vi "CANopencRIOPDODemo.vi"() -> ()   [LabVIEW 2016]
doc: "Write and Read PDO Values for PDO,1 which is mapped to digital values.\nThis example is written for a WAGO 750-307 device."
uses:
  <vilib>/Platform/TimedLoop/XDataNode/timing_clust.ctl
  <vilib>/Platform/TimedLoop/XDataNode/nitl_modes.ctl
  <vilib>/Platform/TimedLoop/XDataNode/wakeup.ctl
  Instance           2 26Saved   CANopencRIOPDODemo .vi
  Instance           3 26Saved   CANopencRIOPDODemo .vi
  <vilib>/FPGAPlugInAG/cRIO-9033/niLvFpga_Close_cRIO-9033.vi
  <vilib>/Platform/TimedLoop/XDataNode/XDataNode.xnode
  <vilib>/rvi/interface/nirviCloseFPGA/nirviCloseFPGA.xnode
  FPGA Bitfiles/EV-MCU_FPGATarget_CANEngine(FPGA)b_eM8Xz3qYJVA.lvbitx
  CAN_Engine(FPGA)_basic.vi
  <vilib>/Platform/TimedLoop/XDataNode/XDNodeRunTimeDep.lvlib
panel:
  out "ID":u32 format="%.0x"
  out "Finished Late? [i-1]":bool
  out "Timing (us)":u32
  out "error out":errorcluster
  in  "Digital Out":bool[](array[boolean])=[FALSE, FALSE, FALSE, FALSE, FALSE, FALSE, FALSE, FALSE, FALSE, FALSE, FALSE, FALSE, FALSE, FALSE, FALSE, FALSE]
  in  "stop":bool
  out "Digital In":bool[](array[boolean])
  # "Project uses 500 Kbaud\nand node ID 1"
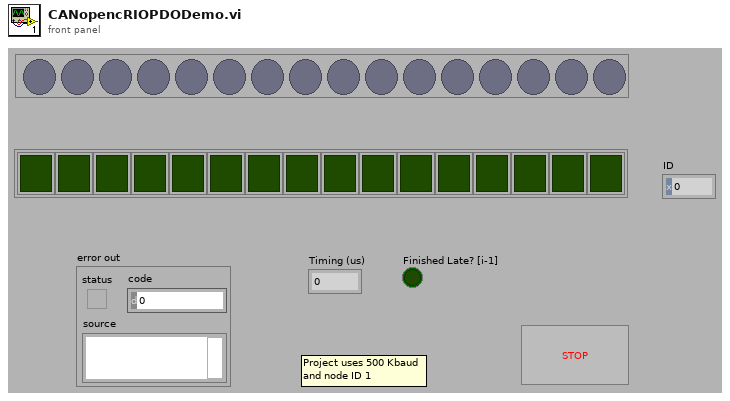
[diagram p1: front panel]
types:
  T1 = enum16{"start remote node", "stop remote node", "reset node", "reset communication", "enter preoperational"}
  T2 = typedef "XDNodeRunTimeDep.lvlib/timing_clust.ctl" = cluster{"Expected End [f-1]":u64, "Actual End [f-1]":u64, "Finished Late? [f-1]":bool, "Expected End [i-1]":u64, "Actual End [i-1]":u64, "Finished Late? [i-1]":bool, "Expected Start [i]":u64, "Actual Start [i]":u64, "Expected Start [f]":u64, "Actual Start [f]":u64, "Source Name":string, "Structure Name":string, "Period":i64, "Deadline":i64, "Offset":i64, "Start":i64, "Priority":i32, "Timeout":i32, "Mode":T3, "Wakeup Reason":T4, "Error":errorcluster, "Source Type":string, "Secondary Source Type":string, "Global End Time":u64, "Global Start Time":u64, "Frame Duration":u64, "Iteration Duration":u64, "Assigned CPU":i32, "I/O Scan Engine Mode":u32}
  T3 = typedef "XDNodeRunTimeDep.lvlib/nitl_modes.ctl" = enum32{"No Change", "Process missed periods, maintain original phase", "Discard missed periods, maintain original phase", "Process missed periods, ignore original phase", "Discard missed periods, ignore original phase"}
  T4 = typedef "XDNodeRunTimeDep.lvlib/wakeup.ctl" = enum32{"Normal", "Aborted", "Asynchronous wakeup", "Timing source error", "Timed loop error", "Timeout"}
  T5 = cluster{"PDO type":enum8{"tx PDO 1", "tx PDO 2", "tx PDO 3", "tx PDO 4"}, "COB ID":u32}
  T6 = cluster{"PDO type":enum8{"rx PDO 1", "rx PDO 2", "rx PDO 3", "rx PDO 4"}, "COB ID":u32}
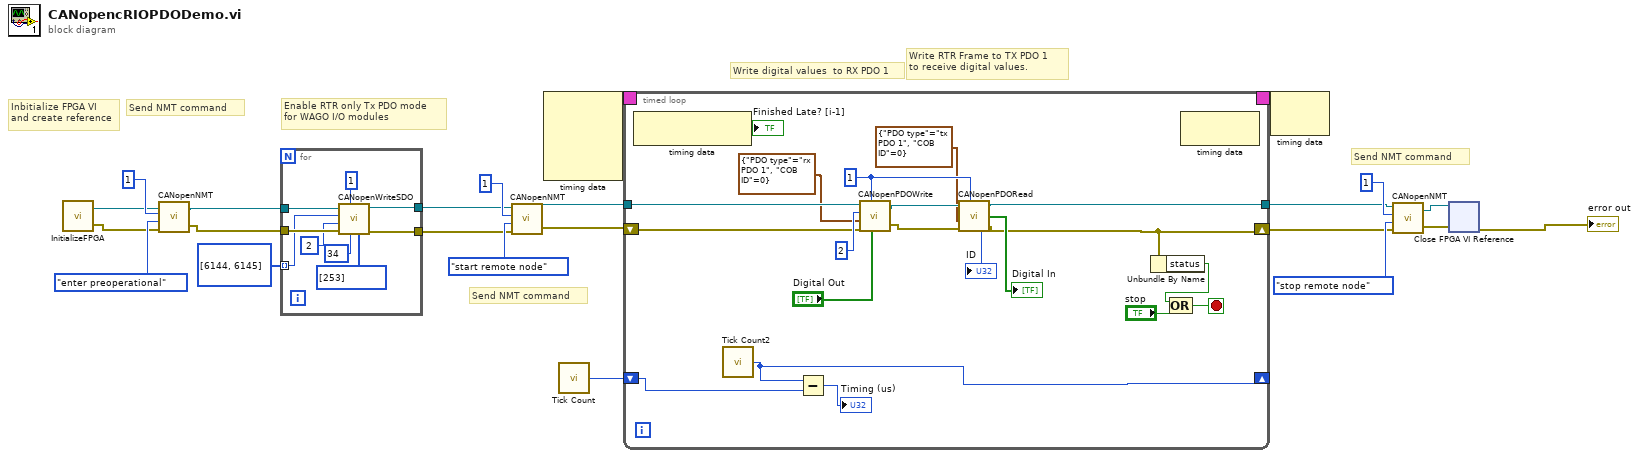
[diagram p0: block diagram]
diagram:
  # "Send NMT command"
  # "Write RTR Frame to TX PDO 1 \nto receive digital values."
  # "Write digital values  to RX PDO 1"
  # "Send NMT command"
  # "Enable RTR only Tx PDO mode\nfor WAGO I/O modules"
  # "Inbitialize FPGA VI \nand create reference"
  # "Send NMT command"
  n1 = call "InitializeFPGA.vi"() -> ("error out"=w12:errorcluster, "FPGA VI Reference Out"=w11:refnum<k20>)  [unwired: 2 in]
  n2 = call "CANopenNMT.vi"("error in"=w12, "Mode"=T1."enter preoperational", "Node ID"=u8 1, "FPGA VI Reference In"=w11) -> ("error out"=w9:errorcluster, "FPGA VI Reference Out"=w10:refnum<k20>)
  n3 = for {
    tunnel: [w32] -> w15
    tunnel: w10 -> [w31]
    tunnel: w9 -> [w30]
    tunnel: [w29] -> w8
    tunnel: u16[] [6144, 6145] -> [w24] mode=indexing
    n4 = call "CANopenWriteSDO.vi"("data array"=u8[] [253], "Byte0 (h40)"=u8 34, "Node ID"=u32 1, "error in"=w30, "Sub Index"=u8 2, "Index"=w24, "FPGA VI Reference In"=w31) -> ("error out"=w32:errorcluster, "FPGA VI Reference Out"=w29:refnum<k20>)  [unwired: 3 in]
  }
  n5 = call "CANopenNMT.vi"("error in"=w15, "Mode"=T1."start remote node", "Node ID"=u8 1, "FPGA VI Reference In"=w8) -> ("error out"=w19:errorcluster, "FPGA VI Reference Out"=w18:refnum<k20>)
  n6 = node-c288() -> (w22:T2)  [unwired: 4 in]
  n7 = call "Tick Count"() -> ("Tick Count(uSec)"=w23:u32)
  n8 = timed-loop {
    tunnel: w18 -> [w46]
    tunnel: [w40] -> w4
    shift-right: [w49] -> _
    shift-left: w23 -> [w50]
    timing: w22 -> [_]
    timing-out: [_] -> w21
    shift-right: [w39] -> w5
    shift-left: w19 -> [w41]
    stop <- w36 stop-if-true
    w35 = u8 1 ("Node ID")
    n9 = node-c288() -> (→"Finished Late? [i-1]":bool)  [unwired: 1 in]
    n10 = call "Tick Count2"() -> ("Tick Count(uSec)"=w49:u32)
    n11 = Subtract(x=w49, y=w50) -> (x-y=→"Timing (us)":u32)
    n12 = call "CANopenPDOWrite.vi"("Boolean In"="Digital Out", "Node ID"=w35, "error in"=w41, "PDO configuration"=T6 {"PDO type"=enum."rx PDO 1", "COB ID"=0}, "DataLength"=u8 2, "FPGA VI Reference In"=w46) -> ("error out"=w45:errorcluster, "FPGA VI Reference Out"=w44:refnum<k20>)
    n13 = call "CANopenPDORead.vi"("FPGA VI Reference In"=w44, "Node ID"=w35, "PDO configuration"=T5 {"PDO type"=enum."tx PDO 1", "COB ID"=0}, "error in"=w45) -> ("ID"=→"ID":u32, "FPGA VI Reference Out"=w40:refnum<k20>, "Boolean array"=→"Digital In":bool[], "error out"=w39:errorcluster)  [unwired: 1 in]
    n14 = Unbundle By Name(w39) -> ("status"=w51:bool)
    n15 = Compound Arithmetic op=OR(w51, "stop") -> (w36:bool)
    n16 = node-c288() -> ()  [unwired: 1 in, 1 out]
  }
  n17 = node-c288(w21) -> ()  [unwired: 1 out]
  n18 = call "CANopenNMT.vi"("error in"=w5, "Mode"=T1."stop remote node", "Node ID"=u8 1, "FPGA VI Reference In"=w4) -> ("error out"=w3:errorcluster, "FPGA VI Reference Out"=w2:refnum<k20>)
  n19 = xnode "Close FPGA VI Reference"("FPGA VI Reference In"=w2, "error in"=w3) -> ("error out"=→"error out":errorcluster)
